vi "_UpdateSpectralPlot.vi"(5 "MassRange# (0)":i32, 6 "MassReference":cluster{"Mass":dbl, "Use":bool}[](array[cluster]), 7 "Current Data":T1={"Scan#"=0, "Run Time (mS)"=0, "TIC X"=[], "TIC Y"=[], "MassRange"=[], "Fixed Mass (amu)"=1.0, "Method"={"StartT(mS)"=0, "#Cycles"=0, "PauseT(uS)"=0, "ScanType"=0, "Polarity"=0, "FixedMass"=0.0, "DelayT(mS)"=0, "Active Ch"=[], "Mass Range"=[]}} {"Method"."Mass Range"."Res" items=["High/High", "Medium/Medium", "Low/Low", "High/Medium", "High/Low", "Medium/High", "Medium/Low", "Low/High", "Low/Medium"]}, 8 "Display Refnum":refnum<vi>) -> ()   [LabVIEW 2015]
uses:
  Type/_Current Data.ctl
  Type/_XML Expt.ctl
  Type/_XML Lens.ctl
  Type/_Mass Range Property.ctl
  Type/_Mass Range Parameters.ctl
  Type/_RT Res Type.ctl
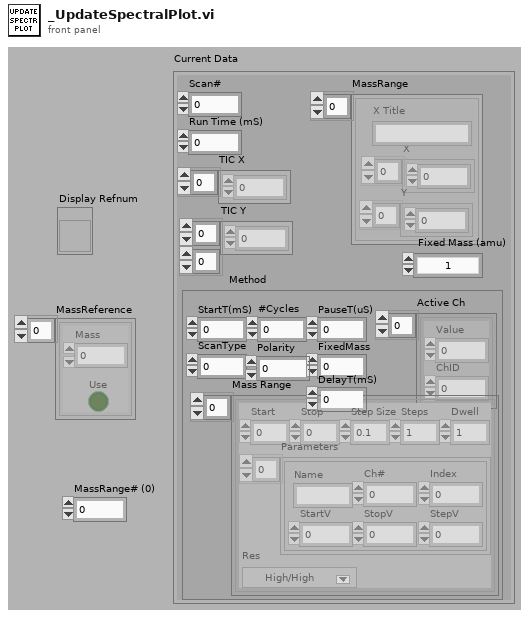
[diagram p1: front panel]
types:
  T1 = typedef "_Current Data.ctl" = cluster{"Scan#":i32, "Run Time (mS)":i32, "TIC X":dbl[], "TIC Y":dbl[][], "MassRange":cluster{"X Title":string, "X":dbl[], "Y":i32[]}[], "Fixed Mass (amu)":dbl, "Method":T2}
  T2 = typedef "_XML Expt.ctl" = cluster{"StartT(mS)":i32, "#Cycles":i32, "PauseT(uS)":i32, "ScanType":i32, "Polarity":u8, "FixedMass":dbl, "DelayT(mS)":i32, "Active Ch":T3[], "Mass Range":T4[]}
  T3 = typedef "_XML Lens.ctl" = cluster{"Value":dbl, "ChID":u8}
  T4 = typedef "_Mass Range Property.ctl" = cluster{"Start":dbl, "Stop":dbl, "Step Size":dbl, "Steps":i32, "Dwell":dbl, "Parameters":T5[], "Res":T6}
  T5 = typedef "_Mass Range Parameters.ctl" = cluster{"Name":string, "Ch#":u8, "StartV":dbl, "StopV":dbl, "StepV":dbl, "Index":u8}
  T6 = typedef "_RT Res Type.ctl" = u16
  T7 = cluster{"X Title":string, "X":dbl[], "Y":i32[]}[]
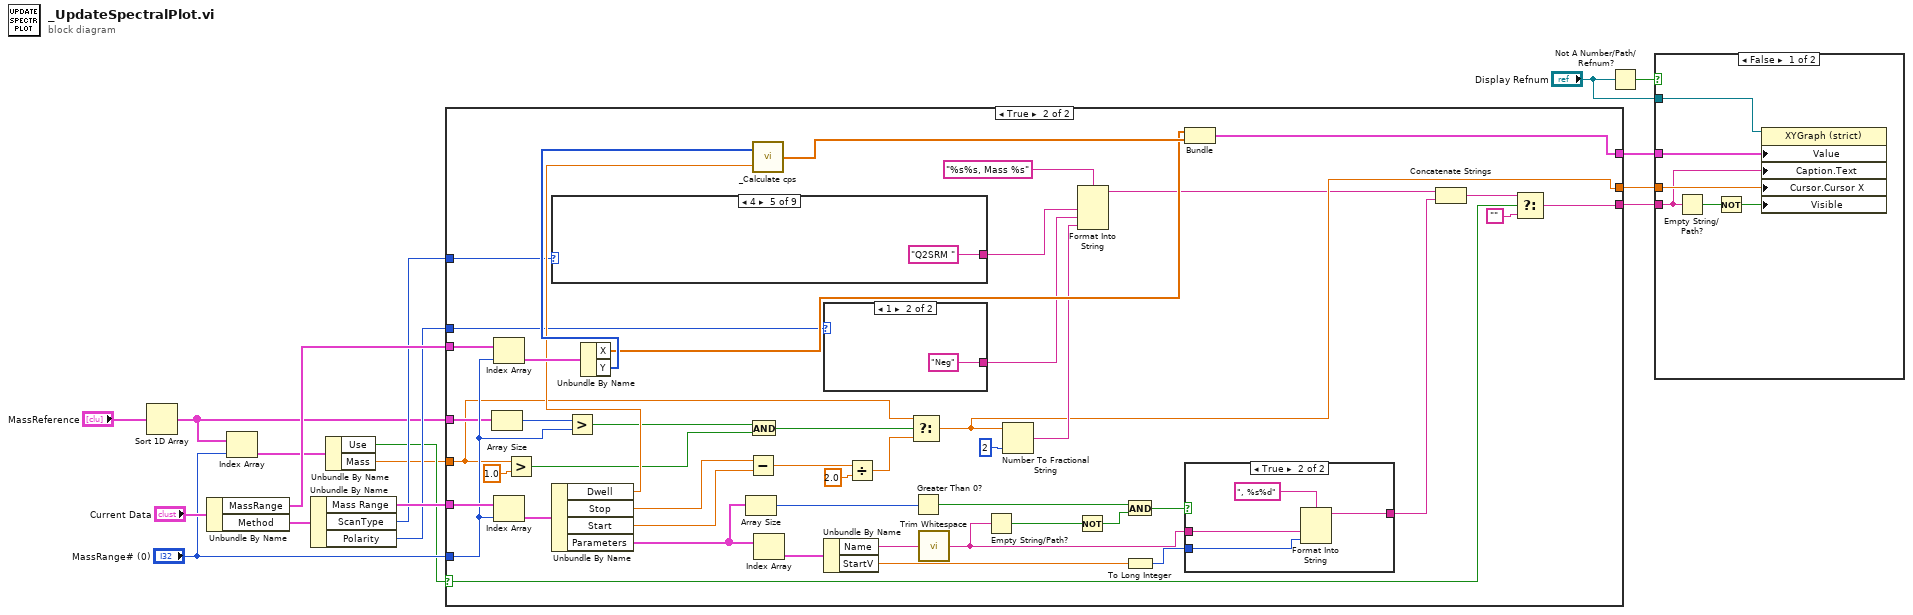
[diagram p0: block diagram]
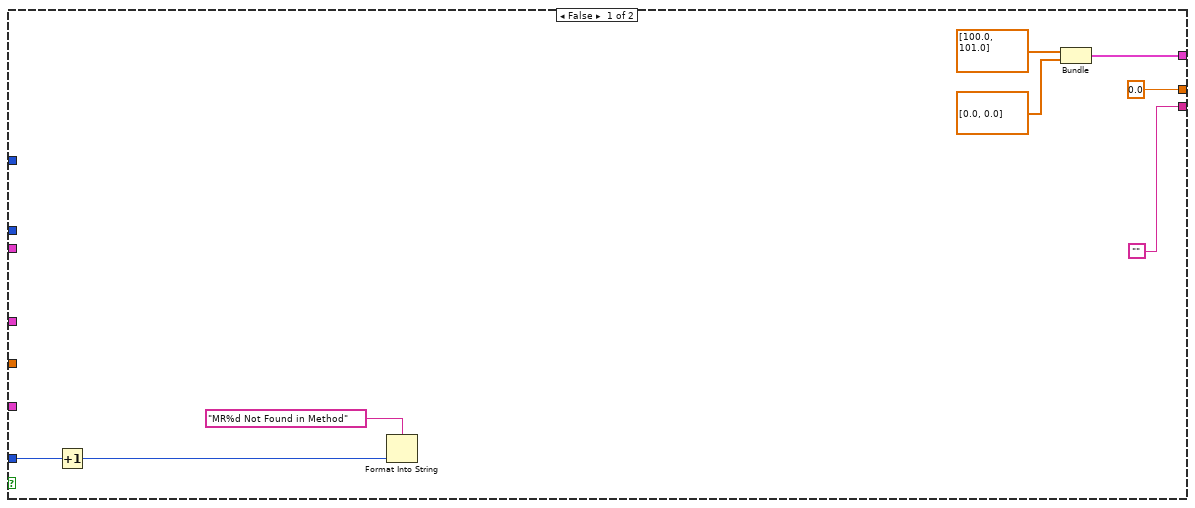
[diagram p3: hidden frame]
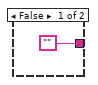
[diagram p4: hidden frame]
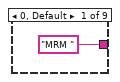
[diagram p5: hidden frame]
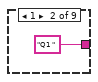
[diagram p6: hidden frame]
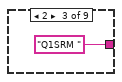
[diagram p7: hidden frame]
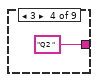
[diagram p8: hidden frame]
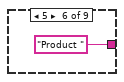
[diagram p9: hidden frame]
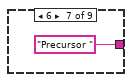
[diagram p10: hidden frame]
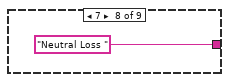
[diagram p11: hidden frame]
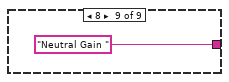
[diagram p12: hidden frame]
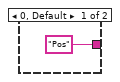
[diagram p13: hidden frame]
diagram:
  n1 = Sort 1D Array(array="MassReference") -> (sorted array=w1:cluster{"Mass":dbl, "Use":bool}[])
  n2 = Unbundle By Name("Current Data") -> ("MassRange"=w15:T7, "Method"=w16:T2)
  n3 = Index Array(array=w1, index="MassRange# (0)") -> (element=w5:cluster{"Mass":dbl, "Use":bool})
  n4 = Unbundle By Name(w16) -> ("Mass Range"=w11:T4[], "ScanType"=w9:i32, "Polarity"=w8:u8)
  n5 = Unbundle By Name(w5) -> ("Use"=w4:bool, "Mass"=w2:dbl)
  n6 = case shown="True" w4 {
    selector: w4 -> [_ w28]
    tunnel: w11 -> [_ w70]
    tunnel: w15 -> [_ w65]
    tunnel: "MassRange# (0)" -> [w22 w51]
    tunnel: [w23 w64] -> w12
    tunnel: ["" w29] -> w10
    tunnel: w9 -> [_ w58]
    tunnel: w8 -> [_ w59]
    tunnel: [0.0 ("Mass") w45] -> w7
    tunnel: w1 -> [_ w27]
    tunnel: w2 -> [_ w26]
    frame False {
      n7 = Increment(x=w22) -> (x+1=w21:i32)
      n8 = Format Into String(format string="MR%d Not Found in Method", w21) -> ()  [unwired: 2 in, 2 out]
      n9 = Bundle(dbl[] [100.0, 101.0], dbl[] [0.0, 0.0]) -> (w23:cluster{dbl[], dbl[]})  [unwired: 1 out]
    }
    frame True {
      n10 = Array Size(array=w27) -> (size(s)=w52:i32)
      n11 = Index Array(array=w65, index=w51) -> (element=w71:cluster{"X Title":string, "X":dbl[], "Y":i32[]})
      n12 = Index Array(array=w70, index=w51) -> (element=w69:T4)
      n13 = Greater?(x=w26, y=1.0) -> (0:w48:bool)
      n14 = case shown="4" w58 {
        tunnel: ["MRM " "Q1 " "Q1SRM " "Q2 " "Q2SRM " "Product " "Precursor " "Neutral Loss " "Neutral Gain "] -> w57
        frame 0, Default {
        }
        frame 1 {
        }
        frame 2 {
        }
        frame 3 {
        }
        frame 4 {
        }
        frame 5 {
        }
        frame 6 {
        }
        frame 7 {
        }
        frame 8 {
        }
      }
      n15 = Unbundle By Name(w69) -> ("Dwell"=w67:dbl, "Stop"=w63:dbl, "Start"=w62:dbl, "Parameters"=w41:T5[])
      n16 = Greater?(x=w52, y=w51) -> (0:w49:bool)
      n17 = Unbundle By Name(w71) -> ("X"=w66:dbl[], "Y"=w68:i32[])
      n18 = Array Size(array=w41) -> (size(s)=w44:i32)
      n19 = Subtract(x=w63, y=w62) -> (x-y=w61:dbl)
      n20 = And(x=w49, y=w48) -> (x .and. y?=w47:bool)
      n21 = call "_Calculate cps.vi"("Dwell (mS)"=w67, "Raw Counts"=w68) -> ("Data in cps"=w72:dbl[])
      n22 = Index Array(array=w41) -> (element=w42:T5)  [unwired: 1 in]
      n23 = case shown="1" w59 {
        tunnel: ["Pos" "Neg"] -> w56
        frame 0, Default {
        }
        frame 1 {
        }
      }
      n24 = Unbundle By Name(w42) -> ("Name"=w40:string, "StartV"=w43:dbl)
      n25 = Divide(x=w61, y=2.0) -> (x/y=w46:dbl)
      n26 = Select(t=w26, s=w47, f=w46) -> (s? t:f=w45:dbl)
      n27 = Greater Than 0?(x=w44) -> (x > 0?=w37:bool)
      n28 = call <vilib>:"Trim Whitespace.vi"("string"=w40) -> ("trimmed string"=w35:string)  [unwired: 1 in]
      n29 = Empty String/Path?(string/path=w35) -> (empty?=w39:bool)
      n30 = Number To Fractional String(number=w45, precision (6)=i16 2) -> (F-format string=w54:string)  [unwired: 2 in]
      n31 = Not(x=w39) -> (.not. x?=w38:bool)
      n32 = Format Into String(format string="%s%s, Mass %s", w57, w56, w54) -> (resulting string=w33:string)  [unwired: 2 in, 1 out]
      n33 = And(x=w37, y=w38) -> (x .and. y?=w36:bool)
      n34 = To Long Integer(number=w43) -> (32bit integer=w34:i32)
      n35 = Bundle("X"=w66, "Data in cps"=w72) -> (w64:cluster{"X":dbl[], "Data in cps":dbl[]})  [unwired: 1 out]
      n36 = case shown="True" w36 {
        tunnel: w35 -> [_ w77]
        tunnel: w34 -> [_ w76]
        tunnel: ["" w74] -> w32
        frame False {
        }
        frame True {
          n37 = Format Into String(format string=", %s%d", w77, w76) -> (resulting string=w74:string)  [unwired: 2 in, 1 out]
        }
      }
      n38 = Concatenate Strings(w33, w32) -> (w31:string)
      n39 = Select(t=w31, s=w28, f="") -> (s? t:f=w29:string)
    }
  }
  n40 = Not A Number/Path/Refnum?(number/path/refnum="Display Refnum") -> (NaN/Path/Refnum?=w14:bool)
  n41 = case shown="False" w14 {
    tunnel: "Display Refnum" -> [w94 _]
    tunnel: w12 -> [w93 _]
    tunnel: w10 -> [w91 _]
    tunnel: w7 -> [w92 _]
    frame False {
      n42 = Empty String/Path?(string/path=w91) -> (empty?=w90:bool)
      n43 = Not(x=w90) -> (.not. x?=w89:bool)
      n44 = property class="XYGraph (strict)"(reference=w94, "Value"=w93, "Caption.Text"=w91, "Cursor.Cursor X"=w92, "Visible"=w89) -> ()  [unwired: 1 in, 2 out]
    }
    frame True {
    }
  }
